vi "F Dwf Digital IO Output Enable Set64.vi"(8 "error in (no error)":errorcluster, 10 "fsOutputEnable":cluster{}, 11 "hdwf":i32) -> (0 "error out":errorcluster, 3 "function return":i32)   [LabVIEW 2019, in "Olasdwf.lvlib"]
doc: "DWFAPI int FDwfDigitalIOOutputEnableSet64(HDWF hdwf, unsigned long long fsOutputEnable);"
uses:
  Olasdwf.lvlib
  Windows/System32/dwf.dll
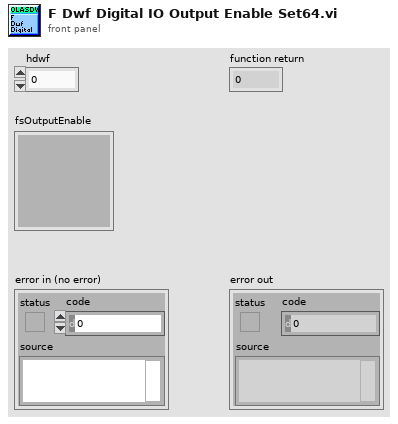
[diagram p1: front panel]
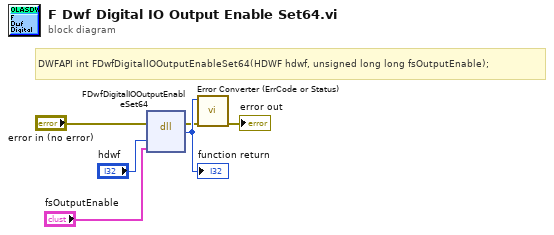
[diagram p0: block diagram]
diagram:
  # "DWFAPI int FDwfDigitalIOOutputEnableSet64(HDWF hdwf, unsigned long long fsOutputEnable);"
  n1 = dll-call lib="C:/Windows/System32/dwf.*" fn="FDwfDigitalIOOutputEnableSet64"(error in="error in (no error)", "hdwf"="hdwf", "fsOutputEnable"="fsOutputEnable") -> (error out=w2:errorcluster, w6:i32)  [unwired: 4 in, 1 out]
  "function return" <- w6
  n2 = call "Error Converter (ErrCode or Status).vi"("error in (no error)"=w2, "error code"=w6) -> ("error out"=→"error out":errorcluster)  [unwired: 9 in]
